vi "MicroPulse - decode IF card sets.vi"(0 "U8":u8[](array[numeric]) format="%.0x") -> (2 "card info":string, 3 "Interface Cards":T1[](array[typedef]) {"FPGA - T" format="%.0f °C"; "Board - T" format="%.0f °C"})   [LabVIEW 2026, in "MicroPulse_Driver.lvlib"]
uses:
  MicroPulse_Driver.lvlib
  Public/Data/Datatypes/MP - interface card status.ctl
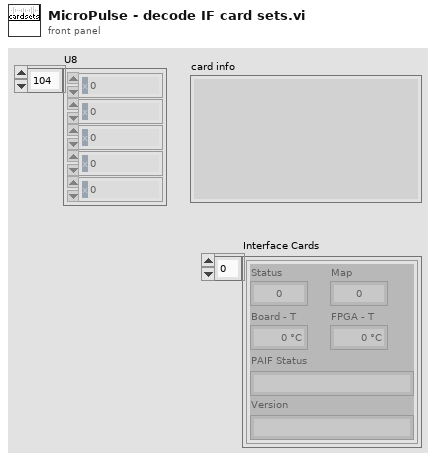
[diagram p1: front panel]
types:
  T1 = typedef "MicroPulse_Driver.lvlib/MP - interface card status.ctl" = cluster{"Status":u8, "Map":u8, "Board - T":u8, "FPGA - T":u8, "PAIF Status":string, "Version":string}
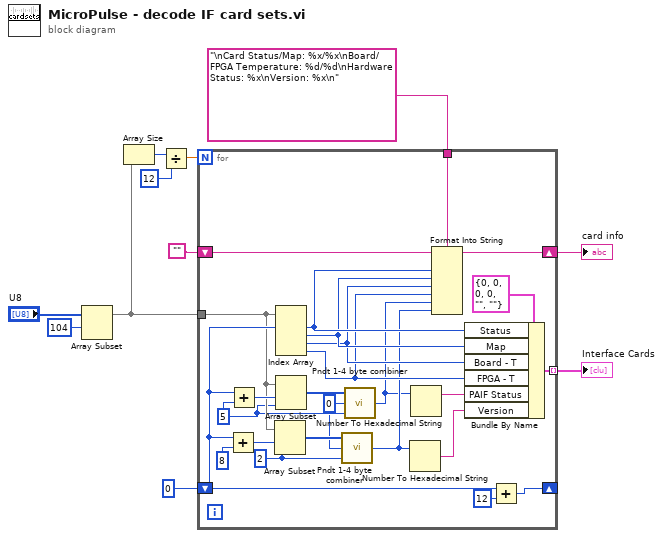
[diagram p0: block diagram]
diagram:
  n1 = Array Subset(array="U8", index=104) -> (w2:u8[])  [unwired: 1 in]
  n2 = Array Size(array=w2) -> (size(s)=w6:i32)
  n3 = Divide(x=w6, y=12) -> (x/y=w4:dbl)
  n4 = for {
    N: w4 -> [_]
    shift-right: [w36] -> _
    shift-left: 0 -> [w29]
    tunnel: w2 -> [w28]
    shift-right: [w22] -> w10
    shift-left: "" -> [w21]
    tunnel: [w32] -> w9 mode=indexing
    tunnel: "\nCard Status/Map: %x/%x\nBoard/FPGA Temperature: %d/%d\nHardware Status: %x\nVersion: %x\n" ("format string") -> [w26]
    w14 = 0 ("start index [0]")
    w20 = 2 ("length")
    w15 = 5 ("y")
    n5 = Add(x=w29, y=8) -> (x+y=w30:i32)
    n6 = Add(x=w29, y=w15) -> (x+y=w33:i32)
    n7 = Array Subset(array=w28, index=w30, length=w20) -> (w19:u8[])
    n8 = Index Array(array=w28, index #1=w29) -> (element #1=w27:u8, element #2=w25:u8, element #3=w24:u8, element #4=w23:u8)  [unwired: 3 in]
    n9 = Array Subset(array=w28, index=w33, length=w15) -> (w16:u8[])
    n10 = call "Pndt 1-4 byte combiner.vi"("#bytes"=w20, "start index [0]"=w14, "[U8] count bytes"=w19) -> ("U32"=w18:u32)
    n11 = call "Pndt 1-4 byte combiner.vi"("#bytes"=w15, "start index [0]"=w14, "[U8] count bytes"=w16) -> ("U32"=w13:u32)
    n12 = Number To Hexadecimal String(2:w18) -> (0:w17:string)  [unwired: 1 in]
    n13 = Number To Hexadecimal String(2:w13) -> (0:w12:string)  [unwired: 1 in]
    n14 = Format Into String(format string=w26, initial string=w21, w27, w25, w24, w23, w13, w18) -> (resulting string=w22:string)  [unwired: 1 in, 1 out]
    n15 = Bundle By Name(cluster=T1 {"Status"=0, "Map"=0, "Board - T"=0, "FPGA - T"=0, "PAIF Status"="", "Version"=""}, "Status"=w27, "Map"=w25, "Board - T"=w24, "FPGA - T"=w23, "PAIF Status"=w12, "Version"=w17) -> (w32:T1)
    n16 = Add(x=w29, y=12) -> (x+y=w36:i32)
  }
  "card info" <- w10
  "Interface Cards" <- w9
